vi "hand-chehao.vi"(0 "Image In":T4, 1 "ROI Descriptor (OCR/OCV 1)":T2={"Global Rectangle"=[253, 103, 559, 182], "Contours"=[{"ID"=enum."External", "Type"=3, "Coordinates"=[253, 103, 559, 182]}]} {"Contours"."Type" items=["No Selection", "Point", "Line", "Rectangle", "Oval", "Polygon", "Freehand Region", "Annulus", "Unused2", "Unused3", "Broken Line", "Freehand Line", "Rotated Rectangle"]}, 2 "File Path (OCR/OCV 1)":path=path "D:/Labviewprogram/视觉/视觉框架/Hand-车牌号.abc", 3 "Parameters (OCR/OCV 1)":T1={"Threshold Data"={"Method"=enum."Uniform", "Looking for"=1, "Color Mode"=0, "Kernel Size"={"Width"=32, "Height"=32}, "Ranges"=[{"Min"=1, "Max"=255}]}, "Reject Border"=TRUE, "Number Of Erosions"=0, "Size & Spacing"={"Segment Algorithm"=0, "Min Bounding Rect Width"=1, "Max Bounding Rect Width"=65536, "Min Bounding Rect Height"=1, "Max Bounding Rect Height"=65536, "Min Character Size"=20, "Max Character Size"=65536, "Min Char Spacing"=1, "Max Horiz Element Spacing"=1, "Max Vert Element Spacing"=0, "Max Space Distance"=65536}, "Read Options"={"Read Strategy"=1, "Read Resolution"=2, "Scale Dependant"=FALSE, "Aspect Ratio"=400, "Acceptance Level"=700, "Substitution Character"="?", "MultiLine"=TRUE}, "Valid Characters"=[], "Use Text Pattern"=FALSE, "Orientation"=0, "# Lines Expected"=0, "Number of Blocks"=4} {"Threshold Data"."Looking for" items=["Light on Dark", "Dark on Light"]; "Threshold Data"."Color Mode" items=["RGB", "HSL", "HSV", "HSI"]; "Size & Spacing"."Segment Algorithm" items=["None", "Shortest Segment", "Legacy Auto Split"]; "Read Options"."Read Strategy" items=["Aggressive", "Conservative"]; "Read Options"."Read Resolution" items=["Low", "Medium", "High"]; "Valid Characters"."Pre-defined characters" items=["Any Character", "User-defined Characters", "Alphabetic", "Alphanumeric", "Uppercase Letters", "Lowercase Letters", "Decimal Digits", "Hexadecimal Digits", "Pattern", "Force Space"]; "Orientation" items=["Baseline inside", "Baseline outside"]}, 7 "error in":errorcluster) -> (20 "Image Out":T4, 21 "String (OCR/OCV 1)":string, 22 "OCR Session (OCR/OCV 1)":T3, 27 "error out":errorcluster)   [LabVIEW 2018]
uses:
  <vilib>/vision/Image Controls.llb/IMAQ Image.ctl
  <vilib>/vision/OCR.llb/IMAQ OCR Session.ctl
  <vilib>/vision/NI_Vision_Development_Module.lvlib
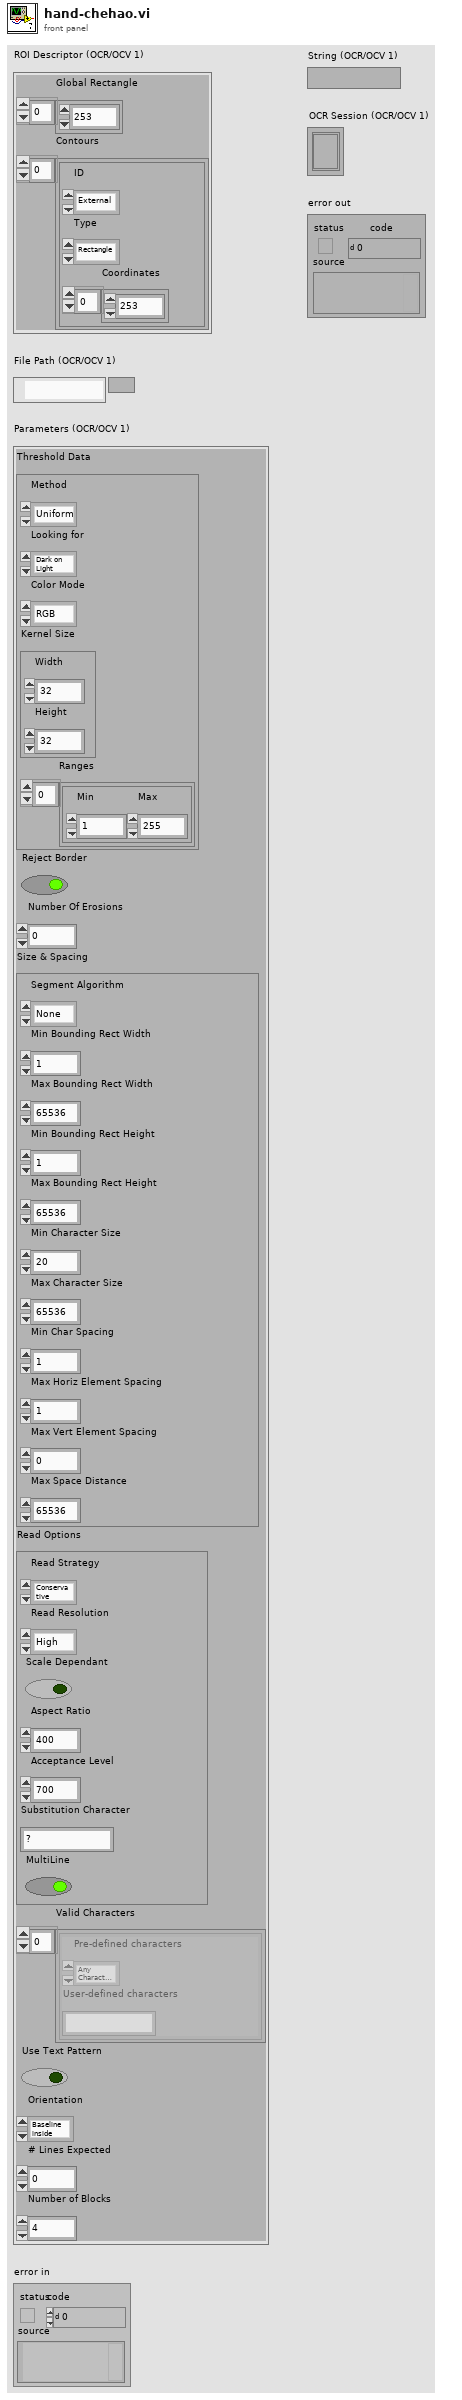
[diagram p1: front panel]
types:
  T1 = cluster{"Threshold Data":cluster{"Method":enum16{"Fixed Range", "Uniform", "Linear", "Non Linear", "Local", "Color"}, "Looking for":u32, "Color Mode":u32, "Kernel Size":cluster{"Width":i32, "Height":i32}, "Ranges":cluster{"Min":i32, "Max":i32}[]}, "Reject Border":bool, "Number Of Erosions":i32, "Size & Spacing":cluster{"Segment Algorithm":u16, "Min Bounding Rect Width":i32, "Max Bounding Rect Width":i32, "Min Bounding Rect Height":i32, "Max Bounding Rect Height":i32, "Min Character Size":i32, "Max Character Size":i32, "Min Char Spacing":i32, "Max Horiz Element Spacing":i32, "Max Vert Element Spacing":i32, "Max Space Distance":i32}, "Read Options":cluster{"Read Strategy":i32, "Read Resolution":i32, "Scale Dependant":bool, "Aspect Ratio":i32, "Acceptance Level":i32, "Substitution Character":string, "MultiLine":bool}, "Valid Characters":cluster{"Pre-defined characters":i32, "User-defined characters":string}[], "Use Text Pattern":bool, "Orientation":u32, "# Lines Expected":u32, "Number of Blocks":i32}
  T2 = cluster{"Global Rectangle":i32[], "Contours":cluster{"ID":enum32{"External", "Internal"}, "Type":u32, "Coordinates":i32[]}[]}
  T3 = typedef "IMAQ OCR Session.ctl" = refnum<k1>
  T4 = typedef "IMAQ Image.ctl" = refnum<image>
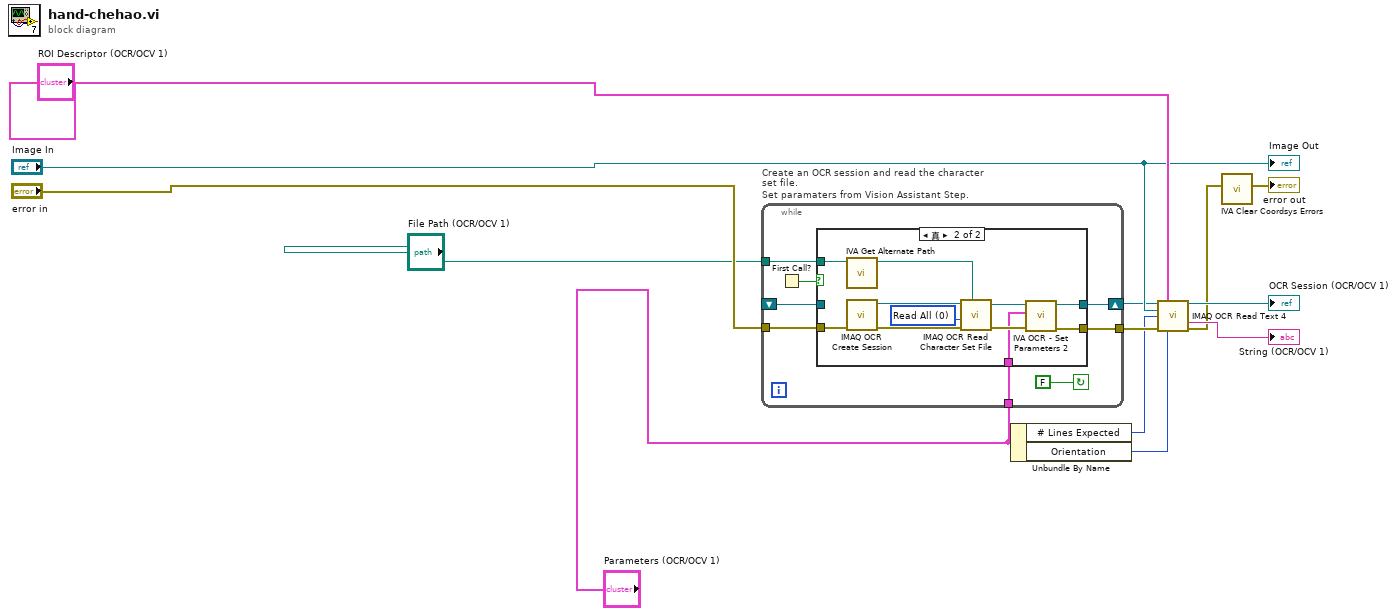
[diagram p0: block diagram]
diagram:
  n1 = while "Create an OCR session and read the character set file.\nSet paramaters from Vision Assistant Step." {
    shift-right: [w18] -> w5
    shift-left: _ -> [w17]
    tunnel: "error in" -> [w20]
    tunnel: "Parameters (OCR/OCV 1)" -> [w16]
    tunnel: "File Path (OCR/OCV 1)" -> [w15]
    tunnel: [w14] -> w6
    stop <- FALSE continue-if-true
    n2 = First Call?() -> (First Call?: T/F=w19:bool)
    n3 = case "条件结构" shown="真" w19 {
      tunnel: w15 -> [_ w27]
      tunnel: w20 -> [w22 w31]
      tunnel: [w23 w29] -> w18
      tunnel: [w22 w28] -> w14
      tunnel: w16 -> [_ w24]
      tunnel: w17 -> [w23 _]
      frame False {
      }
      frame True {
        w32 = 0 items=["Read All", "Read Character Set Only", "Read Properties Only"] ("Read Options")
        n4 = call <vilib>:"IVA Get Alternate Path.vi"("Path In"=w27) -> ("Path Out"=w26:path)  [unwired: 10 out]
        n5 = call "IMAQ OCR Create Session"("error in (no error)"=w31) -> ("error out"=w33:errorcluster, "IMAQ OCR Session"=w34:T3)  [unwired: 9 out]
        n6 = call "IMAQ OCR Read Character Set File"("File Path"=w26, "error in (no error)"=w33, "Read Options"=w32, "IMAQ OCR Session"=w34) -> ("error out"=w30:errorcluster, "IMAQ OCR Session (dup)"=w25:T3)  [unwired: 1 in, 5 out]
        n7 = call <vilib>:"IVA OCR - Set Parameters 2.vi"("error in (no error)"=w30, "Parameters"=w24, "IMAQ OCR Session"=w25) -> ("error out"=w28:errorcluster, "IMAQ OCR Session Out"=w29:T3)  [unwired: 7 in]
      }
    }
  }
  n8 = Unbundle By Name("Parameters (OCR/OCV 1)") -> ("# Lines Expected"=w3:u32, "Orientation"=w4:u32)
  n9 = call "IMAQ OCR Read Text 4"("IMAQ OCR Session"=w5, "ROI Descriptor"="ROI Descriptor (OCR/OCV 1)", "Image"="Image In", "Number of Lines Requested"=w3, "error in (no error)"=w6, "Orientation"=w4) -> ("IMAQ OCR Session (dup)"=→"OCR Session (OCR/OCV 1)":T3, "Read String"=→"String (OCR/OCV 1)":string, "error out"=w2:errorcluster)  [unwired: 7 out]
  n10 = call <vilib>:"IVA Clear Coordsys Errors.vi"("error in (no error)"=w2) -> ("error out"=→"error out":errorcluster)  [unwired: 10 in]
  "Image Out" <- "Image In"
